vi "Is Initialized.vi"(8 "error in":errorcluster, 11 "IMAQdx Base Configure Strategy in":refnum<class "IMAQdx Base Configure Strategy.lvclass">) -> (0 "error out":errorcluster, 2 "Is Initialized?":bool, 3 "IMAQdx Base Configure Strategy out":refnum<class "IMAQdx Base Configure Strategy.lvclass">)   [LabVIEW 2024, in "IMAQdx Base Configure Strategy.lvclass"]
uses:
  IMAQdx Base Configure Strategy.lvclass
  IMAQdx Base Configure Strategy.lvclass/IMAQdx Base Configure Strategy.ctl
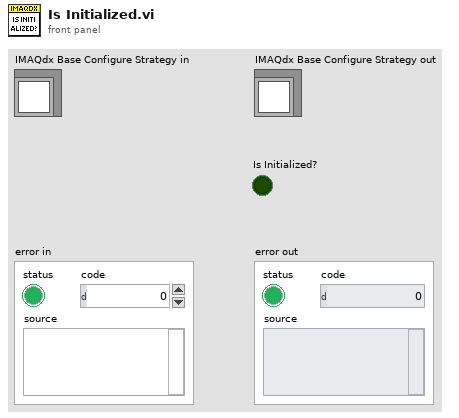
[diagram p1: front panel]
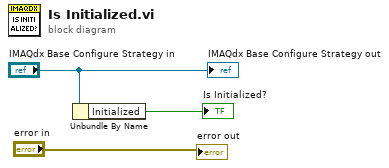
[diagram p0: block diagram]
diagram:
  n1 = Unbundle By Name("IMAQdx Base Configure Strategy in") -> ("Initialized"=→"Is Initialized?":bool)
  "IMAQdx Base Configure Strategy out" <- "IMAQdx Base Configure Strategy in"
  "error out" <- "error in"
